vi "Begin.vi"(8 "error in":errorcluster) -> (0 "error out":errorcluster)   [LabVIEW 2019]
doc: "Called before other user functions, this VI is expected to open initial I/O refnums, load in file data, and do all program initialization. Notice that the <B>error out</B> terminal is simply used for data flow. Wiring it to other structures or subVIs ensures that this VI runs first."
uses:
  <vilib>/Rock Robotics/WPI/SafetyOutput/WPI_SafetyOutputConfigMenu.ctl
  <vilib>/Rock Robotics/WPI/DriverStation/WPI_DriverStationRobotMode2.ctl
  <vilib>/Rock Robotics/WPI/Joystick/WPI_JoystickDeviceEnum.ctl
  <vilib>/Rock Robotics/WPI/ThirdParty/REV Robotics/SPARK MAX/Typedef/Spark MAX Idle Mode.ctl
  <vilib>/Rock Robotics/WPI/ThirdParty/REV Robotics/SPARK MAX/Typedef/Spark MAX Motor Type.ctl
  <vilib>/Rock Robotics/WPI/ThirdParty/Phoenix-LabVIEW/Motor Controller/Controls/CTRE_Phoenix_MotorControl_ControlMode.ctl
  <vilib>/Rock Robotics/WPI/Solenoid/WPI_SolenoidChannel.ctl
  <vilib>/Rock Robotics/SystemInterfaces/DIO/FPGA_DIOChannel.ctl
  <vilib>/Rock Robotics/WPI/Encoder/WPI_EncoderType.ctl
  <vilib>/Rock Robotics/SystemInterfaces/DIO/FPGA_DIORelayChannel.ctl
  <vilib>/Rock Robotics/WPI/Relay/WPI_RelayDirection.ctl
  Robot Global Data.vi
  <vilib>/Rock Robotics/WPI/RobotDrive/WPI_RobotDriveOpen4MotorWithExistingMotors.vi
  <vilib>/Rock Robotics/WPI/Solenoid/WPI_SolenoidOpenDouble.vi
  <vilib>/Rock Robotics/WPI/Switch/WPI_SwitchOpenLimit.vi
  <vilib>/Rock Robotics/WPI/Counter/WPI_CounterDigitalInputToDigitalSource.vi
  <vilib>/Rock Robotics/WPI/Utilities/WPI_GetSetVariantRefNum.vi
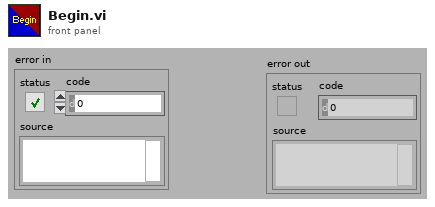
[diagram p1: front panel]
types:
  T1 = typedef "WPI_RelayDirection.ctl" = enum16{"Both directions", "Forward only", "Reverse only"}
  T2 = typedef "FPGA_DIORelayChannel.ctl" = enum8{"Relay 0", "Relay 1", "Relay 2", "Relay 3", "Invalid"}
  T3 = typedef "FPGA_DIOChannel.ctl" = enum8{"DIO 0", "DIO 1", "DIO 2", "DIO 3", "DIO 4", "DIO 5", "DIO 6", "DIO 7", "DIO 8", "DIO 9", "DIO MXP 0", "DIO MXP 1", "DIO MXP 2", "DIO MXP 3", "DIO MXP 4", "DIO MXP 5", "DIO MXP 6", "DIO MXP 7", "DIO MXP 8", "DIO MXP 9", "DIO MXP 10", "DIO MXP 11", "DIO MXP 12", "DIO MXP 13", "DIO MXP 14", "DIO MXP 15", "SPI Port CS1", "SPI Port CS2", "SPI Port CS3", "SPI Port MISO", "SPI Port MOSI", "Invalid"}
  T4 = typedef "WPI_EncoderType.ctl" = enum16{"1x", "2x", "4x"}
  T5 = typedef "WPI_SolenoidChannel.ctl" = enum8{"Solenoid 0", "Solenoid 1", "Solenoid 2", "Solenoid 3", "Solenoid 4", "Solenoid 5", "Solenoid 6", "Solenoid 7", "Invalid"}
  T6 = typedef "CTRE_Phoenix_MotorControl_ControlMode.ctl" = u16
  T7 = typedef "WPI_JoystickDeviceEnum.ctl" = enum16{"USB 0", "USB 1", "USB 2", "USB 3", "USB 4", "USB 5"}
  T8 = typedef "Spark MAX Motor Type.ctl" = enum16{"Brushed", "Brushless"}
  T9 = typedef "Spark MAX Idle Mode.ctl" = enum16{"Coast", "Brake"}
  T10 = typedef "WPI_DriverStationRobotMode2.ctl" = enum16{"Autonomous Disabled", "Autonomous Enabled", "Teleop Disabled", "Teleop Enabled", "Disconnected", "Finish", "Test Disabled", "Test Enabled", "Emergency Stopped"}
  T11 = typedef "WPI_SafetyOutputConfigMenu.ctl" = enum16{"Enable", "Disable"}
  T12 = typedef "WPI_MotorControlDeviceRef.ctl" = cluster{"DeviceStatus":errorcluster, "Type":T13, "PWM":cluster{"PWM Channel":T14, "DeadBand":T15}, "CAN":cluster{"Device Number":u8, "SetOutput VI Ref":variant, "GetOutput VI Ref":variant, "Enable VI Ref":variant, "Disable VI Ref":variant, "Data":variant}, "Invert":bool, "DIO PWM":cluster{"PWM \"Enable\" Channel":T14, "DIOChannel":T3, "PWM Rate":dbl}}
  T13 = typedef "WPI_MotorControlType.ctl" = enum16{"PWM", "CAN", "DIO PWM"}
  T14 = typedef "FPGA_DIOPWMChannel.ctl" = enum8{"PWM 0", "PWM 1", "PWM 2", "PWM 3", "PWM 4", "PWM 5", "PWM 6", "PWM 7", "PWM 8", "PWM 9", "PWM MXP 0", "PWM MXP 1", "PWM MXP 2", "PWM MXP 3", "PWM MXP 4", "PWM MXP 5", "PWM MXP 6", "PWM MXP 7", "PWM MXP 8", "PWM MXP 9", "Invalid"}
  T15 = typedef "WPI_PWMDeadband.ctl" = cluster{"Name":string, "maxPositivePwm":i32, "minPositivePwm":i32, "centerPwm":i32, "maxNegativePwm":i32, "minNegativePwm":i32, "angularRange":u16}
  T16 = typedef "WPI_JoystickDevRef.ctl" = cluster{"Device":T7}
  T17 = typedef "WPI_RobotDriveDevRef.ctl" = cluster{"DevStatus":errorcluster, "Motors[]":T12[], "Square Inputs":bool, "Max Output":dbl}
  T18 = typedef "WPI_SolenoidDevRef.ctl" = cluster{"DevStatus":errorcluster, "Pneumatics Control Module":u8, "Forward Solenoid Channel":T5, "Reverse Solenoid Channel":T5}
  T19 = typedef "WPI_SwitchDevRef.ctl" = cluster{"DevStatus":errorcluster, "DIO Channel":T3, "CntIndex":T20, "Normally Closed":bool}
  T20 = typedef "FPGA_CounterCtrSystemIndex.ctl" = enum8{"Ctr 0", "Ctr 1", "Ctr 2", "Ctr 3", "Ctr 4", "Ctr 5", "Ctr 6", "Ctr 7", "Invalid"}
  T21 = typedef "WPI_RelayDevRef.ctl" = cluster{"DevStatus":errorcluster, "Relay Channel":T2, "Relay Direction":T1}
  T22 = typedef "WPI_CompressorDevRef.ctl" = cluster{"DevStatus":errorcluster, "Pneumatics Control Module":u8}
  T23 = typedef "WPI_DigitalInputDevRef.ctl" = cluster{"DevStatus":errorcluster, "DIO Channel":T3}
  T24 = typedef "FPGA_CounterEncoderSourceConvertionLVSourceType.ctl" = cluster{"DevStatus":errorcluster, "AnalogTriggerMode?":bool, "DigitalMode":cluster{"DIO Channel":T25}, "AnalogTriggerMode":cluster{"AnalogTriggerIndex":T26, "OutputType":T27}}
  T25 = typedef "FPGA_DIODigitalSourceChannel.ctl" = enum8{"DIO 0", "DIO 1", "DIO 2", "DIO 3", "DIO 4", "DIO 5", "DIO 6", "DIO 7", "DIO 8", "DIO 9", "DIO MXP 0", "DIO MXP 1", "DIO MXP 2", "DIO MXP 3", "DIO MXP 4", "DIO MXP 5", "DIO MXP 6", "DIO MXP 7", "DIO MXP 8", "DIO MXP 9", "DIO MXP 10", "DIO MXP 11", "DIO MXP 12", "DIO MXP 13", "DIO MXP 14", "DIO MXP 15", "SPI Port CS1", "SPI Port CS2", "SPI Port CS3", "SPI Port MISO", "SPI Port MOSI", "Disabled"}
  T26 = typedef "FPGA_AnalogTriggerIndex.ctl" = enum8{"Trig 0", "Trig 1", "Trig 2", "Trig 3", "Trig 4", "Trig 5", "Trig 6", "Trig 7", "Invalid"}
  T27 = typedef "FPGA_AnalogTriggerOutType.ctl" = enum16{"InWindow", "TriggerState", "Rising", "Falling"}
  T28 = typedef "WPI_EncoderDevRef.ctl" = cluster{"DevStatus":errorcluster, "EncoderIndex":T29, "CounterIndex":T20, "DistancePerCount":dbl, "Decoding Type":T4}
  T29 = typedef "FPGA_EncoderIdx.ctl" = enum8{"Enc 0", "Enc 1", "Enc 2", "Enc 3", "Enc 4", "Enc 5", "Enc 6", "Enc 7", "Invalid"}
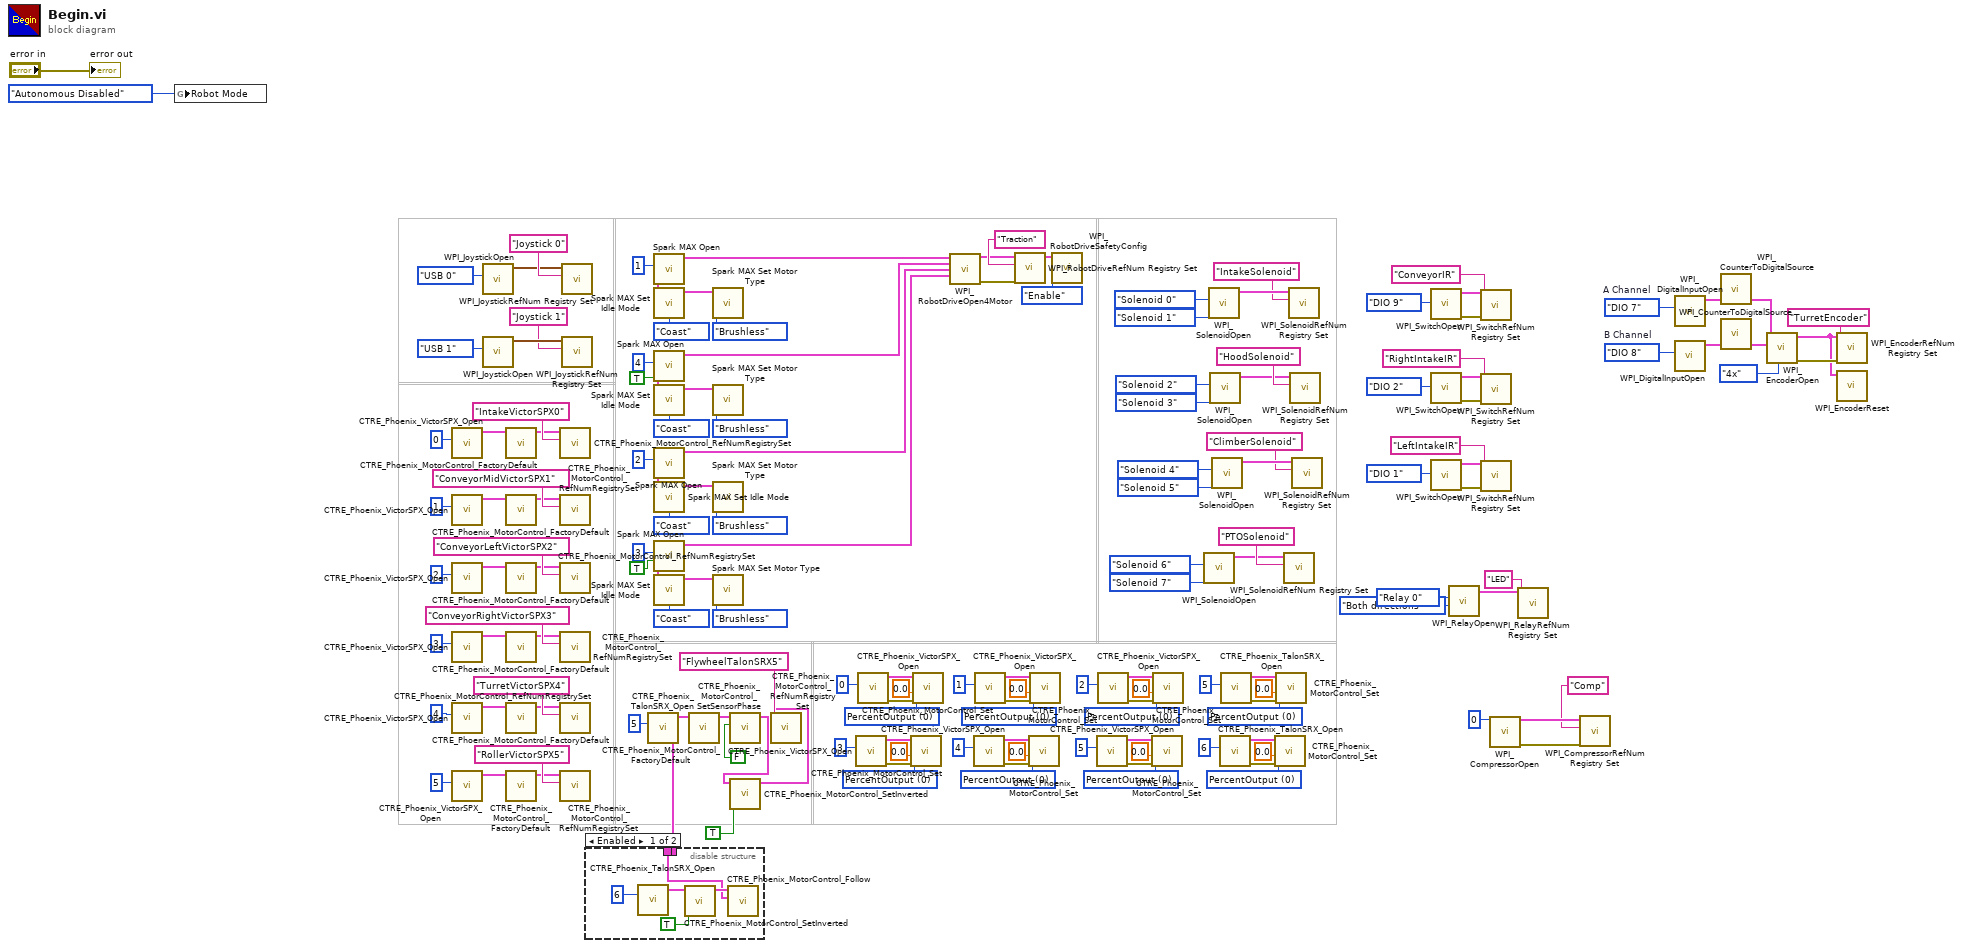
[diagram p0: block diagram]
diagram:
  w30 = FPGA_DIOChannel."DIO 8"  # B Channel
  w29 = FPGA_DIOChannel."DIO 7"  # A Channel
  w52 = T6 0 items=["PercentOutput"=0, "Position"=1, "Velocity"=2, "Current"=3, "Follower"=5, "MotionProfile"=6, "MotionMagic"=7, "MotionMagicArc"=8, "MotionProfileArc"=10, "Disabled"=15] ("Control Mode")
  w53 = T6 0 items=["PercentOutput"=0, "Position"=1, "Velocity"=2, "Current"=3, "Follower"=5, "MotionProfile"=6, "MotionMagic"=7, "MotionMagicArc"=8, "MotionProfileArc"=10, "Disabled"=15] ("Control Mode")
  w63 = T6 0 items=["PercentOutput"=0, "Position"=1, "Velocity"=2, "Current"=3, "Follower"=5, "MotionProfile"=6, "MotionMagic"=7, "MotionMagicArc"=8, "MotionProfileArc"=10, "Disabled"=15] ("Control Mode")
  w62 = T6 0 items=["PercentOutput"=0, "Position"=1, "Velocity"=2, "Current"=3, "Follower"=5, "MotionProfile"=6, "MotionMagic"=7, "MotionMagicArc"=8, "MotionProfileArc"=10, "Disabled"=15] ("Control Mode")
  w72 = T6 0 items=["PercentOutput"=0, "Position"=1, "Velocity"=2, "Current"=3, "Follower"=5, "MotionProfile"=6, "MotionMagic"=7, "MotionMagicArc"=8, "MotionProfileArc"=10, "Disabled"=15] ("Control Mode")
  w73 = T6 0 items=["PercentOutput"=0, "Position"=1, "Velocity"=2, "Current"=3, "Follower"=5, "MotionProfile"=6, "MotionMagic"=7, "MotionMagicArc"=8, "MotionProfileArc"=10, "Disabled"=15] ("Control Mode")
  w82 = T6 0 items=["PercentOutput"=0, "Position"=1, "Velocity"=2, "Current"=3, "Follower"=5, "MotionProfile"=6, "MotionMagic"=7, "MotionMagicArc"=8, "MotionProfileArc"=10, "Disabled"=15] ("Control Mode")
  w115 = T6 0 items=["PercentOutput"=0, "Position"=1, "Velocity"=2, "Current"=3, "Follower"=5, "MotionProfile"=6, "MotionMagic"=7, "MotionMagicArc"=8, "MotionProfileArc"=10, "Disabled"=15] ("Control Mode")
  n1 = global write "Robot Global Data.vi" "Robot Mode"(WPI_DriverStationRobotMode2."Autonomous Disabled" ("Robot Mode")) -> ()
  n2 = call <vilib>:"CTRE_Phoenix_VictorSPX_Open.vi"("Device Number"=u8 0) -> ("CAN Talon SRX Ref"=w97:T12)  [unwired: 9 in, 1 out]
  n3 = call <vilib>:"CTRE_Phoenix_VictorSPX_Open.vi"("Device Number"=u8 1) -> ("CAN Talon SRX Ref"=w95:T12)  [unwired: 9 in, 1 out]
  n4 = call <vilib>:"CTRE_Phoenix_VictorSPX_Open.vi"("Device Number"=u8 2) -> ("CAN Talon SRX Ref"=w94:T12)  [unwired: 9 in, 1 out]
  n5 = call <vilib>:"CTRE_Phoenix_VictorSPX_Open.vi"("Device Number"=u8 3) -> ("CAN Talon SRX Ref"=w90:T12)  [unwired: 9 in, 1 out]
  n6 = call <vilib>:"CTRE_Phoenix_VictorSPX_Open.vi"("Device Number"=u8 4) -> ("CAN Talon SRX Ref"=w92:T12)  [unwired: 9 in, 1 out]
  n7 = call <vilib>:"CTRE_Phoenix_VictorSPX_Open.vi"("Device Number"=u8 5) -> ("CAN Talon SRX Ref"=w87:T12)  [unwired: 9 in, 1 out]
  n8 = call <vilib>:"WPI_JoystickOpen.vi"("JoystickDevice"=WPI_JoystickDeviceEnum."USB 0") -> ("JoystickDevRef"=w148:T16)  [unwired: 10 in]
  n9 = call <vilib>:"WPI_JoystickOpen.vi"("JoystickDevice"=WPI_JoystickDeviceEnum."USB 1") -> ("JoystickDevRef"=w109:T16)  [unwired: 10 in]
  n10 = call <vilib>:"CTRE_Phoenix_MotorControl_FactoryDefault.vi"("PhoenixMotorControlDevRef"=w97) -> ("PhoenixMotorControlDevRef"=w96:T12)  [unwired: 9 in, 1 out]
  n11 = call <vilib>:"CTRE_Phoenix_MotorControl_FactoryDefault.vi"("PhoenixMotorControlDevRef"=w95) -> ("PhoenixMotorControlDevRef"=w91:T12)  [unwired: 9 in, 1 out]
  n12 = call <vilib>:"CTRE_Phoenix_MotorControl_FactoryDefault.vi"("PhoenixMotorControlDevRef"=w94) -> ("PhoenixMotorControlDevRef"=w89:T12)  [unwired: 9 in, 1 out]
  n13 = call <vilib>:"CTRE_Phoenix_MotorControl_FactoryDefault.vi"("PhoenixMotorControlDevRef"=w90) -> ("PhoenixMotorControlDevRef"=w93:T12)  [unwired: 9 in, 1 out]
  n14 = call <vilib>:"CTRE_Phoenix_MotorControl_FactoryDefault.vi"("PhoenixMotorControlDevRef"=w92) -> ("PhoenixMotorControlDevRef"=w88:T12)  [unwired: 9 in, 1 out]
  n15 = call <vilib>:"CTRE_Phoenix_MotorControl_FactoryDefault.vi"("PhoenixMotorControlDevRef"=w87) -> ("PhoenixMotorControlDevRef"=w86:T12)  [unwired: 9 in, 1 out]
  n16 = call <vilib>:"CTRE_Phoenix_MotorControl_RefNumRegistrySet.vi"("refnum name"="IntakeVictorSPX0", "PhoenixMotorControlDevRef"=w96) -> ()  [unwired: 8 in, 2 out]
  n17 = call <vilib>:"CTRE_Phoenix_MotorControl_RefNumRegistrySet.vi"("refnum name"="ConveyorMidVictorSPX1", "PhoenixMotorControlDevRef"=w91) -> ()  [unwired: 8 in, 2 out]
  n18 = call <vilib>:"CTRE_Phoenix_MotorControl_RefNumRegistrySet.vi"("refnum name"="ConveyorLeftVictorSPX2", "PhoenixMotorControlDevRef"=w89) -> ()  [unwired: 8 in, 2 out]
  n19 = call <vilib>:"CTRE_Phoenix_MotorControl_RefNumRegistrySet.vi"("refnum name"="ConveyorRightVictorSPX3", "PhoenixMotorControlDevRef"=w93) -> ()  [unwired: 8 in, 2 out]
  n20 = call <vilib>:"CTRE_Phoenix_MotorControl_RefNumRegistrySet.vi"("refnum name"="TurretVictorSPX4", "PhoenixMotorControlDevRef"=w88) -> ()  [unwired: 8 in, 2 out]
  n21 = call <vilib>:"CTRE_Phoenix_MotorControl_RefNumRegistrySet.vi"("refnum name"="RollerVictorSPX5", "PhoenixMotorControlDevRef"=w86) -> ()  [unwired: 8 in, 2 out]
  n22 = call <vilib>:"WPI_JoystickRefNum Registry Set.vi"("refnum name"="Joystick 0", "JoystickDevRef"=w148) -> ()  [unwired: 8 in, 2 out]
  n23 = call <vilib>:"WPI_JoystickRefNum Registry Set.vi"("refnum name"="Joystick 1", "JoystickDevRef"=w109) -> ()  [unwired: 8 in, 2 out]
  n24 = call <vilib>:"CTRE_Phoenix_TalonSRX_Open.vi"("Device Number"=u8 5) -> ("CAN Talon SRX Ref"=w12:T12)  [unwired: 9 in, 1 out]
  n25 = disable-structure shown="Enabled" {
    disable-tunnel: w12 -> [_ _]
    disable-tunnel: w12 -> [w155 _]
    frame Enabled {
      n26 = call <vilib>:"CTRE_Phoenix_TalonSRX_Open.vi"("Device Number"=u8 6) -> ("CAN Talon SRX Ref"=w157:T12)  [unwired: 9 in, 1 out]
      n27 = call <vilib>:"CTRE_Phoenix_MotorControl_SetInverted.vi"("Invert?"=TRUE, "PhoenixMotorControlDevRef"=w157) -> ("PhoenixMotorControlDevRef"=w156:T12)  [unwired: 8 in, 1 out]
      n28 = call <vilib>:"CTRE_Phoenix_MotorControl_Follow.vi"("Master Controller to Follow"=w155, "PhoenixMotorControlDevRef"=w156) -> ()  [unwired: 8 in, 2 out]
    }
    frame Disabled {
    }
  }
  n29 = call <vilib>:"Spark MAX Open.vi"("Device Number"=u8 1) -> ("MotorControlDeviceRef"=w127:T12)  [unwired: 9 in, 1 out]
  n30 = call <vilib>:"Spark MAX Set Idle Mode.vi"("Idle Mode"=Spark_MAX_Idle_Mode."Coast", "MotorControlDeviceRef in"=w127) -> ("MotorControlDeviceRef out"=w140:T12)  [unwired: 8 in, 1 out]
  n31 = call <vilib>:"Spark MAX Open.vi"("Invert"=TRUE, "Device Number"=u8 4) -> ("MotorControlDeviceRef"=w126:T12)  [unwired: 8 in, 1 out]
  n32 = call <vilib>:"Spark MAX Set Idle Mode.vi"("Idle Mode"=Spark_MAX_Idle_Mode."Coast", "MotorControlDeviceRef in"=w126) -> ("MotorControlDeviceRef out"=w139:T12)  [unwired: 8 in, 1 out]
  n33 = call <vilib>:"Spark MAX Open.vi"("Device Number"=u8 2) -> ("MotorControlDeviceRef"=w125:T12)  [unwired: 9 in, 1 out]
  n34 = call <vilib>:"Spark MAX Set Idle Mode.vi"("Idle Mode"=Spark_MAX_Idle_Mode."Coast", "MotorControlDeviceRef in"=w125) -> ("MotorControlDeviceRef out"=w132:T12)  [unwired: 8 in, 1 out]
  n35 = call <vilib>:"Spark MAX Open.vi"("Invert"=TRUE, "Device Number"=u8 3) -> ("MotorControlDeviceRef"=w124:T12)  [unwired: 8 in, 1 out]
  n36 = call <vilib>:"Spark MAX Set Idle Mode.vi"("Idle Mode"=Spark_MAX_Idle_Mode."Coast", "MotorControlDeviceRef in"=w124) -> ("MotorControlDeviceRef out"=w131:T12)  [unwired: 8 in, 1 out]
  n37 = call <vilib>:"CTRE_Phoenix_MotorControl_FactoryDefault.vi"("PhoenixMotorControlDevRef"=w12) -> ("PhoenixMotorControlDevRef"=w85:T12)  [unwired: 9 in, 1 out]
  n38 = call <vilib>:"Spark MAX Set Motor Type.vi"("Motor Type"=Spark_MAX_Motor_Type."Brushless", "MotorControlDevRef"=w140) -> ()  [unwired: 8 in, 2 out]
  n39 = call <vilib>:"Spark MAX Set Motor Type.vi"("Motor Type"=Spark_MAX_Motor_Type."Brushless", "MotorControlDevRef"=w139) -> ()  [unwired: 8 in, 2 out]
  n40 = call <vilib>:"Spark MAX Set Motor Type.vi"("Motor Type"=Spark_MAX_Motor_Type."Brushless", "MotorControlDevRef"=w132) -> ()  [unwired: 8 in, 2 out]
  n41 = call <vilib>:"Spark MAX Set Motor Type.vi"("Motor Type"=Spark_MAX_Motor_Type."Brushless", "MotorControlDevRef"=w131) -> ()  [unwired: 8 in, 2 out]
  n42 = call <vilib>:"CTRE_Phoenix_MotorControl_SetSensorPhase.vi"("PhaseSensor"=FALSE, "PhoenixMotorControlDevRef"=w85) -> ("PhoenixMotorControlDevRef"=w11:T12)  [unwired: 8 in, 1 out]
  n43 = call <vilib>:"CTRE_Phoenix_MotorControl_SetInverted.vi"("Invert?"=TRUE, "PhoenixMotorControlDevRef"=w11) -> ("PhoenixMotorControlDevRef"=w10:T12)  [unwired: 8 in, 1 out]
  n44 = call <vilib>:"CTRE_Phoenix_MotorControl_RefNumRegistrySet.vi"("refnum name"="FlywheelTalonSRX5", "PhoenixMotorControlDevRef"=w10) -> ()  [unwired: 8 in, 2 out]
  n45 = call <vilib>:"CTRE_Phoenix_VictorSPX_Open.vi"("Device Number"=u8 3) -> ("error out"=w78:errorcluster, "CAN Talon SRX Ref"=w79:T12)  [unwired: 9 in]
  n46 = call <vilib>:"CTRE_Phoenix_VictorSPX_Open.vi"("Device Number"=u8 0) -> ("error out"=w119:errorcluster, "CAN Talon SRX Ref"=w118:T12)  [unwired: 9 in]
  n47 = call <vilib>:"CTRE_Phoenix_MotorControl_Set.vi"("error in (no error)"=w78, "Output"=0.0, "Control Mode"=w82, "PhoenixMotorControlDevRef"=w79) -> ()  [unwired: 6 in, 2 out]
  n48 = call <vilib>:"CTRE_Phoenix_MotorControl_Set.vi"("error in (no error)"=w119, "Output"=0.0, "Control Mode"=w115, "PhoenixMotorControlDevRef"=w118) -> ()  [unwired: 6 in, 2 out]
  n49 = call-poly <vilib>:"WPI_RobotDriveOpen4Motor.vi"("Rear Left Motor Dev Ref"=w127, "Rear Right Motor Dev Ref"=w126, "Front Left Motor Dev Ref"=w125, "Front Right Motor Dev Ref"=w124) -> ("RobotDriveDevRef"=w144:T17, "error out"=w145:errorcluster)  [unwired: 10 in]
  n50 = call <vilib>:"CTRE_Phoenix_VictorSPX_Open.vi"("Device Number"=u8 4) -> ("error out"=w68:errorcluster, "CAN Talon SRX Ref"=w69:T12)  [unwired: 9 in]
  n51 = call <vilib>:"CTRE_Phoenix_VictorSPX_Open.vi"("Device Number"=u8 1) -> ("error out"=w77:errorcluster, "CAN Talon SRX Ref"=w76:T12)  [unwired: 9 in]
  n52 = call <vilib>:"WPI_RobotDriveRefNum Registry Set.vi"("error in (no error)"=w145, "refnum name"="Traction", "RobotDriveDevRef"=w144) -> ("RobotDriveDevRef"=w152:T17)  [unwired: 1 in, 7 out]
  n53 = call <vilib>:"CTRE_Phoenix_MotorControl_Set.vi"("error in (no error)"=w68, "Output"=0.0, "Control Mode"=w72, "PhoenixMotorControlDevRef"=w69) -> ()  [unwired: 6 in, 2 out]
  n54 = call <vilib>:"CTRE_Phoenix_MotorControl_Set.vi"("error in (no error)"=w77, "Output"=0.0, "Control Mode"=w73, "PhoenixMotorControlDevRef"=w76) -> ()  [unwired: 6 in, 2 out]
  n55 = call <vilib>:"WPI_RobotDriveSafetyConfig.vi"("mode"=WPI_SafetyOutputConfigMenu."Enable", "RobotDriveDevRef"=w152) -> ()  [unwired: 8 in, 2 out]
  n56 = call <vilib>:"CTRE_Phoenix_VictorSPX_Open.vi"("Device Number"=u8 5) -> ("error out"=w67:errorcluster, "CAN Talon SRX Ref"=w66:T12)  [unwired: 9 in]
  n57 = call <vilib>:"CTRE_Phoenix_VictorSPX_Open.vi"("Device Number"=u8 2) -> ("error out"=w58:errorcluster, "CAN Talon SRX Ref"=w59:T12)  [unwired: 9 in]
  n58 = call <vilib>:"CTRE_Phoenix_MotorControl_Set.vi"("error in (no error)"=w67, "Output"=0.0, "Control Mode"=w63, "PhoenixMotorControlDevRef"=w66) -> ()  [unwired: 6 in, 2 out]
  n59 = call <vilib>:"CTRE_Phoenix_MotorControl_Set.vi"("error in (no error)"=w58, "Output"=0.0, "Control Mode"=w62, "PhoenixMotorControlDevRef"=w59) -> ()  [unwired: 6 in, 2 out]
  n60 = call-poly <vilib>:"WPI_SolenoidOpen.vi"("Reverse Solenoid Channel"=WPI_SolenoidChannel."Solenoid 7", "Forward Solenoid Channel"=WPI_SolenoidChannel."Solenoid 6") -> ("SolenoidDevRef"=w37:T18)  [unwired: 8 in, 1 out]
  n61 = call-poly <vilib>:"WPI_SolenoidOpen.vi"("Reverse Solenoid Channel"=WPI_SolenoidChannel."Solenoid 1", "Forward Solenoid Channel"=WPI_SolenoidChannel."Solenoid 0") -> ("SolenoidDevRef"=w112:T18)  [unwired: 8 in, 1 out]
  n62 = call-poly <vilib>:"WPI_SolenoidOpen.vi"("Reverse Solenoid Channel"=WPI_SolenoidChannel."Solenoid 3", "Forward Solenoid Channel"=WPI_SolenoidChannel."Solenoid 2") -> ("SolenoidDevRef"=w45:T18)  [unwired: 8 in, 1 out]
  n63 = call-poly <vilib>:"WPI_SolenoidOpen.vi"("Reverse Solenoid Channel"=WPI_SolenoidChannel."Solenoid 5", "Forward Solenoid Channel"=WPI_SolenoidChannel."Solenoid 4") -> ("SolenoidDevRef"=w40:T18)  [unwired: 8 in, 1 out]
  n64 = call <vilib>:"CTRE_Phoenix_TalonSRX_Open.vi"("Device Number"=u8 6) -> ("error out"=w48:errorcluster, "CAN Talon SRX Ref"=w49:T12)  [unwired: 9 in]
  n65 = call <vilib>:"CTRE_Phoenix_TalonSRX_Open.vi"("Device Number"=u8 5) -> ("error out"=w57:errorcluster, "CAN Talon SRX Ref"=w56:T12)  [unwired: 9 in]
  n66 = call <vilib>:"CTRE_Phoenix_MotorControl_Set.vi"("error in (no error)"=w48, "Output"=0.0, "Control Mode"=w52, "PhoenixMotorControlDevRef"=w49) -> ()  [unwired: 6 in, 2 out]
  n67 = call <vilib>:"CTRE_Phoenix_MotorControl_Set.vi"("error in (no error)"=w57, "Output"=0.0, "Control Mode"=w53, "PhoenixMotorControlDevRef"=w56) -> ()  [unwired: 6 in, 2 out]
  n68 = call <vilib>:"WPI_SolenoidRefNum Registry Set.vi"("refnum name"="PTOSolenoid", "SolenoidDevRef"=w37) -> ()  [unwired: 8 in, 2 out]
  n69 = call <vilib>:"WPI_SolenoidRefNum Registry Set.vi"("refnum name"="IntakeSolenoid", "SolenoidDevRef"=w112) -> ()  [unwired: 8 in, 2 out]
  n70 = call <vilib>:"WPI_SolenoidRefNum Registry Set.vi"("refnum name"="HoodSolenoid", "SolenoidDevRef"=w45) -> ()  [unwired: 8 in, 2 out]
  n71 = call <vilib>:"WPI_SolenoidRefNum Registry Set.vi"("refnum name"="ClimberSolenoid", "SolenoidDevRef"=w40) -> ()  [unwired: 8 in, 2 out]
  n72 = call-poly <vilib>:"WPI_SwitchOpen.vi"("DIO Channel"=FPGA_DIOChannel."DIO 9") -> ("error out"=w34:errorcluster, "SwitchDevRef"=w33:T19)  [unwired: 9 in]
  n73 = call-poly <vilib>:"WPI_SwitchOpen.vi"("DIO Channel"=FPGA_DIOChannel."DIO 2") -> ("error out"=w13:errorcluster, "SwitchDevRef"=w14:T19)  [unwired: 9 in]
  n74 = call-poly <vilib>:"WPI_SwitchOpen.vi"("DIO Channel"=FPGA_DIOChannel."DIO 1") -> ("error out"=w20:errorcluster, "SwitchDevRef"=w19:T19)  [unwired: 9 in]
  n75 = call <vilib>:"WPI_RelayOpen.vi"("Relay Direction"=WPI_RelayDirection."Both directions", "Relay Channel"=FPGA_DIORelayChannel."Relay 0") -> ("RelayDevRef"=w4:T21)  [unwired: 8 in, 1 out]
  n76 = call <vilib>:"WPI_SwitchRefNum Registry Set.vi"("error in (no error)"=w34, "refnum name"="ConveyorIR", "SwitchDevRef"=w33) -> ()  [unwired: 7 in, 2 out]
  n77 = call <vilib>:"WPI_SwitchRefNum Registry Set.vi"("error in (no error)"=w13, "refnum name"="RightIntakeIR", "SwitchDevRef"=w14) -> ()  [unwired: 7 in, 2 out]
  n78 = call <vilib>:"WPI_SwitchRefNum Registry Set.vi"("error in (no error)"=w20, "refnum name"="LeftIntakeIR", "SwitchDevRef"=w19) -> ()  [unwired: 7 in, 2 out]
  n79 = call <vilib>:"WPI_CompressorOpen.vi"("Pneumatics Control Module (0)"=u8 0) -> ("CompressorDevRef"=w7:T22, "error out"=w6:errorcluster)  [unwired: 13 in]
  n80 = call <vilib>:"WPI_RelayRefNum Registry Set.vi"("refnum name"="LED", "RelayDevRef"=w4) -> ()  [unwired: 8 in, 2 out]
  n81 = call <vilib>:"WPI_CompressorRefNum Registry Set.vi"("error in (no error)"=w6, "refnum name"="Comp", "CompressorDevRef"=w7) -> ()  [unwired: 7 in, 2 out]
  n82 = call <vilib>:"WPI_DigitalInputOpen.vi"("DIO Channel"=w29) -> ("DigitalInputDevRef"=w26:T23)  [unwired: 1 in, 9 out]
  n83 = call <vilib>:"WPI_DigitalInputOpen.vi"("DIO Channel"=w30) -> ("DigitalInputDevRef"=w27:T23)  [unwired: 1 in, 9 out]
  n84 = call-poly <vilib>:"WPI_CounterToDigitalSource.vi"("DigitalInputDevRef"=w26) -> ("Digital Source"=w25:T24)  [unwired: 6 out]
  n85 = call-poly <vilib>:"WPI_CounterToDigitalSource.vi"("DigitalInputDevRef"=w27) -> ("Digital Source"=w28:T24)  [unwired: 6 out]
  n86 = call <vilib>:"WPI_EncoderOpen.vi"("Decoding Type"=WPI_EncoderType."4x", "BSource"=w28, "ASource"=w25) -> ("error out"=w24:errorcluster, "EncoderDevRef"=w21:T28)  [unwired: 5 in, 2 out]
  n87 = call <vilib>:"WPI_EncoderRefNum Registry Set.vi"("error in (no error)"=w24, "refnum name"="TurretEncoder", "EncoderDevRef"=w21) -> ()  [unwired: 7 in, 2 out]
  n88 = call <vilib>:"WPI_EncoderReset.vi"("EncoderDevRef"=w21) -> ()  [unwired: 9 in, 2 out]
  "error out" <- "error in"
